vi "C4If_openDevice.vi"(0 "c4if in":refnum<k24>, 5 "devNo in":i64, 11 "error in (no error)":errorcluster) -> (4 "c4if out":refnum<k24>, 6 "c4dev out":refnum<k24>, 15 "error out":errorcluster)   [LabVIEW 2015, in "libC4HdlLV.lvlib"]
uses:
  libC4HdlLV.lvlib
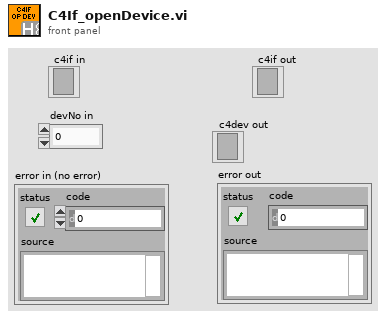
[diagram p1: front panel]
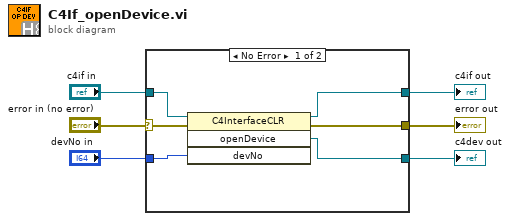
[diagram p0: block diagram]
diagram:
  n1 = case shown="No Error" "error in (no error)" {
    selector: "error in (no error)" -> [w12 w14]
    tunnel: [w9 w14] -> w6
    tunnel: [w8 _] -> w2
    tunnel: "c4if in" -> [w11 w13]
    tunnel: [w7 w13] -> w3
    tunnel: "devNo in" -> [w10 _]
    frame No Error {
      n2 = invoke class="C4InterfaceCLR" method="openDevice"(reference=w11, error in=w12, "devNo"=w10) -> (reference out=w7:refnum<k24>, error out=w9:errorcluster, "openDevice"=w8:refnum<k24>)  [unwired: 1 in, 1 out]
    }
    frame Error {
    }
  }
  "error out" <- w6
  "c4if out" <- w3
  "c4dev out" <- w2
